vi "Save_dialogue_dose_Q.vi"() -> (3 "output 1":dbl)   [LabVIEW 2013]
panel:
  in  "Накопленная доза":string="1"
  in  "OK Button":bool
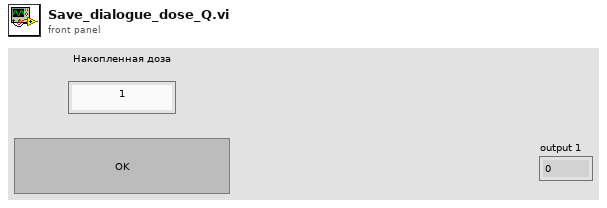
[diagram p1: front panel]
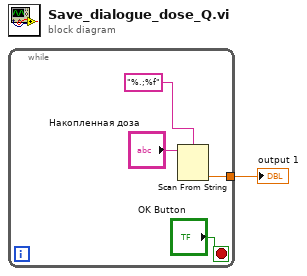
[diagram p0: block diagram]
diagram:
  n1 = while {
    tunnel: [w2] -> w1
    stop <- "OK Button" stop-if-true
    n2 = Scan From String(format string="%.;%f", input string="Накопленная доза") -> (output 1=w2:dbl)  [unwired: 3 in, 3 out]
  }
  "output 1" <- w1
